vi "station4_bit to array.vi"(8 "error in (no error)":errorcluster, 11 "ST1_Controls_from_PLC":i64[](array[numeric])=[0, 0, 0, 0, 0]) -> (0 "error out":errorcluster, 2 "1 on state":i32[](array[numeric]), 3 "1 result array":bool[](array[boolean]))   [LabVIEW 2017]
panel:
  out "cycle rslt":bool
  out "HB st1":bool
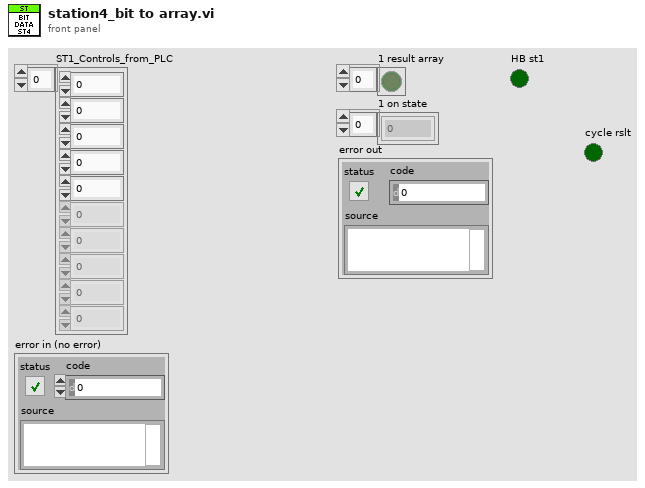
[diagram p1: front panel]
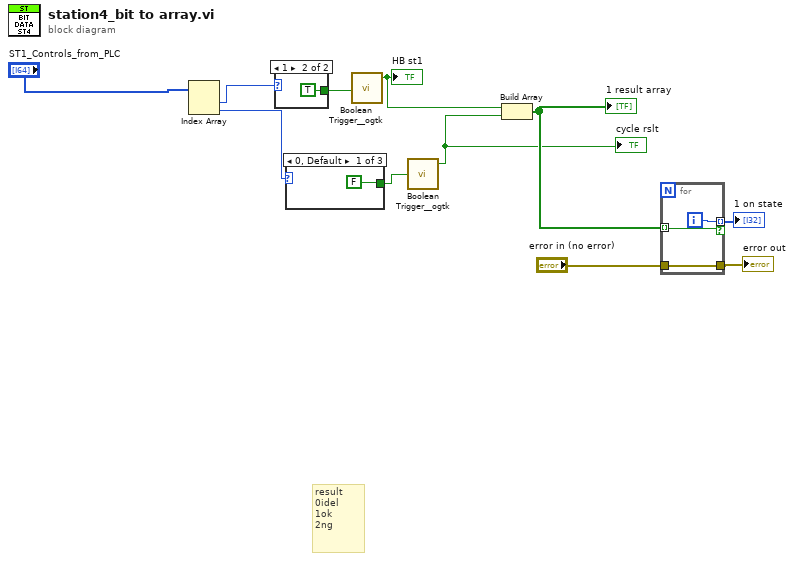
[diagram p0: block diagram]
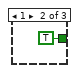
[diagram p2: hidden frame]
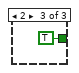
[diagram p3: hidden frame]
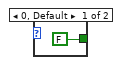
[diagram p4: hidden frame]
diagram:
  # "result\n0idel\n1ok\n2ng"
  n1 = Index Array(array="ST1_Controls_from_PLC") -> (element #1=w11:i64, element #2=w1:i64)  [unwired: 2 in]
  n2 = case shown="1" w11 {
    tunnel: [FALSE TRUE] -> w9
    frame 0, Default {
    }
    frame 1 {
    }
  }
  n3 = case shown="0, Default" w1 {
    tunnel: [FALSE TRUE TRUE] -> w10
    frame 0, Default {
    }
    frame 1 {
    }
    frame 2 {
    }
  }
  n4 = call <userlib>:"Boolean Trigger__ogtk.vi"("Boolean Input"=w9) -> ("Rising Edge"=w7:bool)  [unwired: 1 in, 1 out]
  "HB st1" <- w7
  n5 = call <userlib>:"Boolean Trigger__ogtk.vi"("Boolean Input"=w10) -> ("Rising Edge"=w2:bool)  [unwired: 1 in, 1 out]
  "cycle rslt" <- w2
  n6 = Build Array(w7, w2) -> (w6:bool[])
  "1 result array" <- w6
  n7 = for {
    tunnel: [w19] -> w5 mode=indexing if=w17
    tunnel: "error in (no error)" -> [w18]
    tunnel: [w18] -> w4
    tunnel: w6 -> [w17] mode=indexing
    i -> [w19]
  }
  "1 on state" <- w5
  "error out" <- w4
